vi "Build Installed Folder Paths.vi"() -> (2 "Application Folder Path":path, 3 "Data Folder Path":path)   [LabVIEW 2024, in "SEECD System Explorer.lvlib"]
uses:
  SEECD System Explorer.lvlib
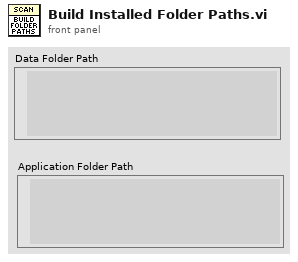
[diagram p1: front panel]
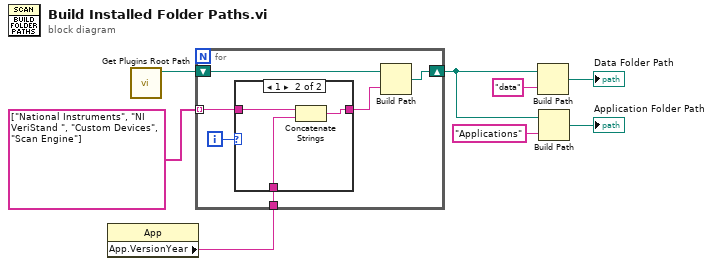
[diagram p0: block diagram]
diagram:
  n1 = property class="App"() -> ("App.VersionYear"=w7:string)  [unwired: 2 in, 2 out]
  n2 = call "Get Plugins Root Path.vi"() -> ("plugins root path"=w1:path)  [unwired: 10 in, 1 out]
  n3 = for {
    shift-right: [w13] -> w5
    shift-left: w1 -> [w14]
    tunnel: string[] ["National Instruments", "NI VeriStand ", "Custom Devices", "Scan Engine"] -> [w10] mode=indexing
    tunnel: w7 -> [w9]
    i -> [w12]
    n4 = case shown="1" w12 {
      tunnel: [w15 w17] -> w11
      tunnel: w10 -> [w15 w18]
      tunnel: w9 -> [_ w16]
      frame Default {
      }
      frame 1 {
        n5 = Concatenate Strings(w18, w16) -> (w17:string)
      }
    }
    n6 = Build Path(base path=w14, name or relative path=w11) -> (appended path=w13:path)
  }
  n7 = Build Path(base path=w5, name or relative path="data") -> (appended path=→"Data Folder Path":path)
  n8 = Build Path(base path=w5, name or relative path="Applications") -> (appended path=→"Application Folder Path":path)
